vi "Get EEPROM Array.vi"(8 "error in (no error)":errorcluster, 10 "Unique FRU Input":T1, 11 "CSV Path":path) -> (0 "error out":errorcluster, 2 "EEPROM Array":u8[](array[numeric]) format="%02x")   [LabVIEW 2016]
doc: "Get the EEPROM Unmodified array from CSV, then replace it with the FRU Written Bytes"
uses:
  Type Definitions/Unique FRU Input.ctl
  Type Definitions/FRU Type.ctl
  <vilib>/Utility/file.llb/Read Delimited Spreadsheet (string).vi
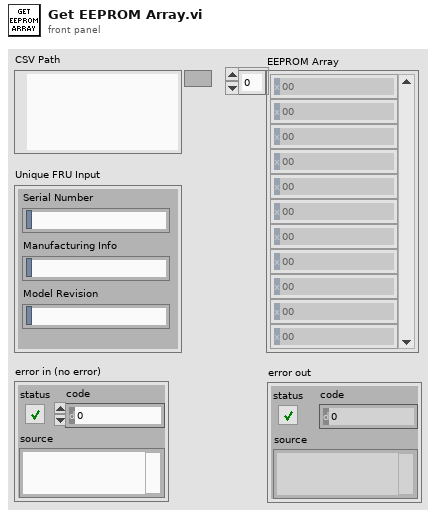
[diagram p1: front panel]
types:
  T1 = typedef "Unique FRU Input.ctl" = cluster{"Serial Number":string, "Manufacturing Info":string, "Model Revision":string}
  T2 = typedef "FRU Type.ctl" = enum16{"FRU Initialized", "EEROM Write Protect", "EEPROM Version", "ADI Data Set (Ph-2 GUI)", "Manufacturer's Name", "Product Name", "Serial Number", "Manufacturing Info", "Model Revision", "Alarm Enable", "SCM Internal Temp Limit", "SCM Average Percentage Temp Limit", "PSU1 Iout Limit", "PSU1 Internal Temp Limit", "PSU1 Vin High Limit", "PSU1 Vin Low Limit", "PSU1 Average Percentage Iout Limit", "PSU2 Iout Limit", "PSU2 Internal Temp Limit", "PSU2 Vin High Limit", "PSU2 Vin Low Limit", "PSU2 Average Percentage Iout Limit", "EEPROM Unmodified"}
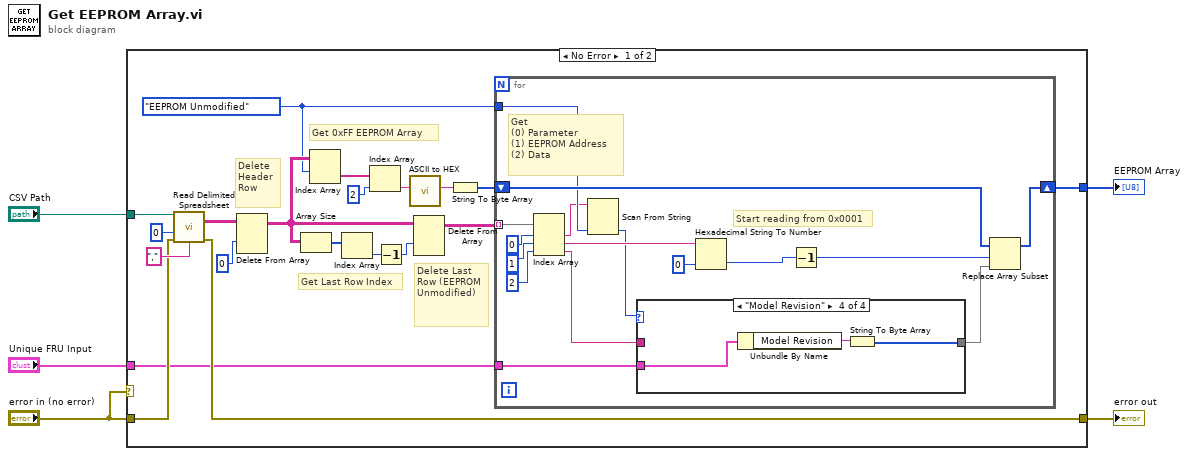
[diagram p0: block diagram]
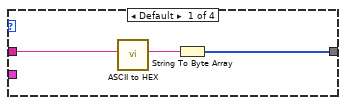
[diagram p2: hidden frame]
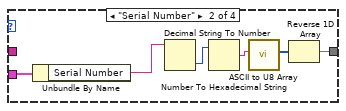
[diagram p3: hidden frame]
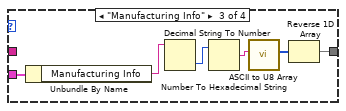
[diagram p4: hidden frame]
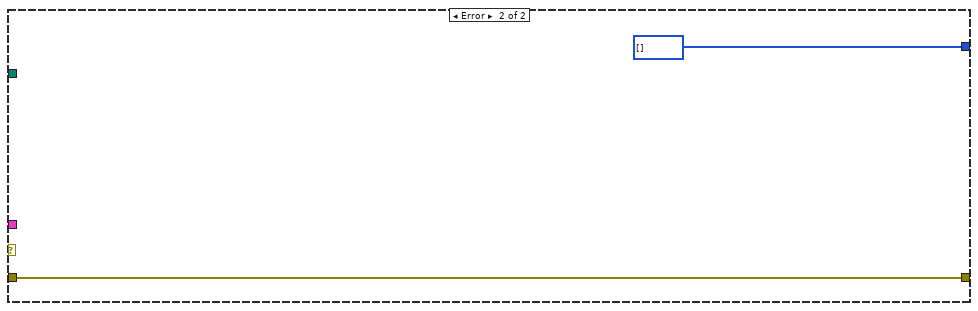
[diagram p5: hidden frame]
diagram:
  n1 = case shown="No Error" "error in (no error)" {
    tunnel: "CSV Path" -> [w23 _]
    tunnel: "error in (no error)" -> [w21 w61]
    tunnel: [w22 w61] -> w4
    tunnel: [w13 u8[] [] ("unsigned byte array")] -> w1
    tunnel: "Unique FRU Input" -> [w6 _]
    frame No Error {
      w7 = FRU_Type."EEPROM Unmodified" ("FRU Type")
      # "Get Last Row Index"
      # "Delete Last Row (EEPROM Unmodified)"
      # "Get 0xFF EEPROM Array"
      # "Delete Header Row"
      n2 = call-poly <vilib>:"Read Delimited Spreadsheet.vi"("file path (dialog if empty)"=w23, "start of read offset (chars.:0)"=0, "error in (no error)"=w21, "delimiter (\\t)"="," ("delimiter (\\t)")) -> ("all rows"=w20:string[][], "error out"=w22:errorcluster)  [unwired: 6 in, 4 out]
      n3 = Delete From Array(array=w20, index (row)=0) -> (array with subset deleted=w12:string[][])  [unwired: 2 in, 1 out]
      n4 = Array Size(array=w12) -> (size(s)=w11:i32[])
      n5 = Index Array(array=w12, index (row)=w7) -> (element=w17:string[])  [unwired: 1 in]
      n6 = Index Array(array=w11) -> (element=w9:i32)  [unwired: 1 in]
      n7 = Index Array(array=w17, index=2) -> (element=w16:string)
      n8 = Decrement(x=w9) -> (x-1=w8:i32)
      n9 = call "ASCII to HEX.vi"("ASCII String"=w16) -> ("Hex String"=w15:string)  [unwired: 10 in]
      n10 = Delete From Array(array=w12, index (row)=w8) -> (array with subset deleted=w10:string[][])  [unwired: 2 in, 1 out]
      n11 = String To Byte Array(string=w15) -> (unsigned byte array=w14:u8[])
      n12 = for {
        tunnel: w10 -> [w41] mode=indexing
        shift-right: [w26] -> w13
        shift-left: w14 -> [w37]
        tunnel: w7 -> [w32]
        tunnel: w6 -> [w29]
        # "Start reading from 0x0001"
        # "Get\n(0) Parameter\n(1) EEPROM Address \n(2) Data"
        n13 = Index Array(array=w41, index #1=0 ("index"), index #2=1 ("index"), index #3=2 ("index")) -> (element #1=w31:string, element #2=w33:string, element #3=w27:string)
        n14 = Scan From String(input string=w31, default 1=w32) -> (output 1=w30:T2)  [unwired: 3 in, 3 out]
        n15 = case shown="\"Model Revision\"" w30 {
          tunnel: [w43 w48 w54 w59] -> w28
          tunnel: w29 -> [_ w47 w53 w57]
          tunnel: w27 -> [w42 _ _ _]
          frame Default {
            n16 = call "ASCII to HEX.vi"("ASCII String"=w42) -> ("Hex String"=w44:string)  [unwired: 10 in]
            n17 = String To Byte Array(string=w44) -> (unsigned byte array=w43:u8[])
          }
          frame "Serial Number" {
            n18 = Unbundle By Name(w47) -> ("Serial Number"=w46:string)
            n19 = Decimal String To Number(string=w46) -> (number=w50:i32)  [unwired: 2 in, 1 out]
            n20 = Number To Hexadecimal String(2:w50) -> (0:w45:string)  [unwired: 1 in]
            n21 = call "ASCII to U8 Array.vi"("ASCII String"=w45) -> ("U8 Array"=w49:u8[])  [unwired: 10 in]
            n22 = Reverse 1D Array(array=w49) -> (reversed array=w48:u8[])
          }
          frame "Manufacturing Info" {
            n23 = Unbundle By Name(w53) -> ("Manufacturing Info"=w52:string)
            n24 = Decimal String To Number(string=w52) -> (number=w56:i32)  [unwired: 2 in, 1 out]
            n25 = Number To Hexadecimal String(2:w56) -> (0:w51:string)  [unwired: 1 in]
            n26 = call "ASCII to U8 Array.vi"("ASCII String"=w51) -> ("U8 Array"=w55:u8[])  [unwired: 10 in]
            n27 = Reverse 1D Array(array=w55) -> (reversed array=w54:u8[])
          }
          frame "Model Revision" {
            n28 = Unbundle By Name(w57) -> ("Model Revision"=w58:string)
            n29 = String To Byte Array(string=w58) -> (unsigned byte array=w59:u8[])
          }
        }
        n30 = Hexadecimal String To Number(string=w33, default (0uL)=0) -> (number=w39:i32)  [unwired: 1 in, 1 out]
        n31 = Decrement(x=w39) -> (x-1=w38:i32)
        n32 = Replace Array Subset(array=w37, new element=w28, index=w38) -> (w26:u8[])
      }
    }
    frame Error {
    }
  }
  "error out" <- w4
  "EEPROM Array" <- w1
